vi "Scripting_SaveVi.vi"(7 "ForceResaving(False)":bool, 8 "error in (no error)":errorcluster, 10 "NewPath":path, 11 "VIRefToSaveIn":refnum<vi>) -> (0 "error out":errorcluster, 3 "VIRefToSaveOut":refnum<vi>)   [LabVIEW 2020]
uses:
  SubVIs/GOOP_ProductType.ctl
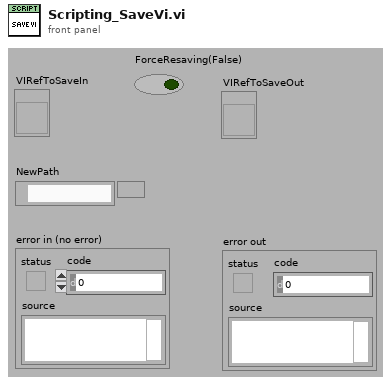
[diagram p1: front panel]
types:
  T1 = typedef "GOOP_ProductType.ctl" = enum16{"InvalidType", "Community Edition", "Professional Edition", "UML Community Edition", "UML Architect Edition"}
  T2 = enum32{"invalid lock state", "Not Locked", "Locked (No Password)", "Password-protected"}
  T3 = enum32{"invalid VI type", "Standard VI", "Control VI", "Global VI", "Polymorphic VI", "Configuration VI", "SubSystem", "Facade VI", "Method VI", "Statechart Diagram VI"}
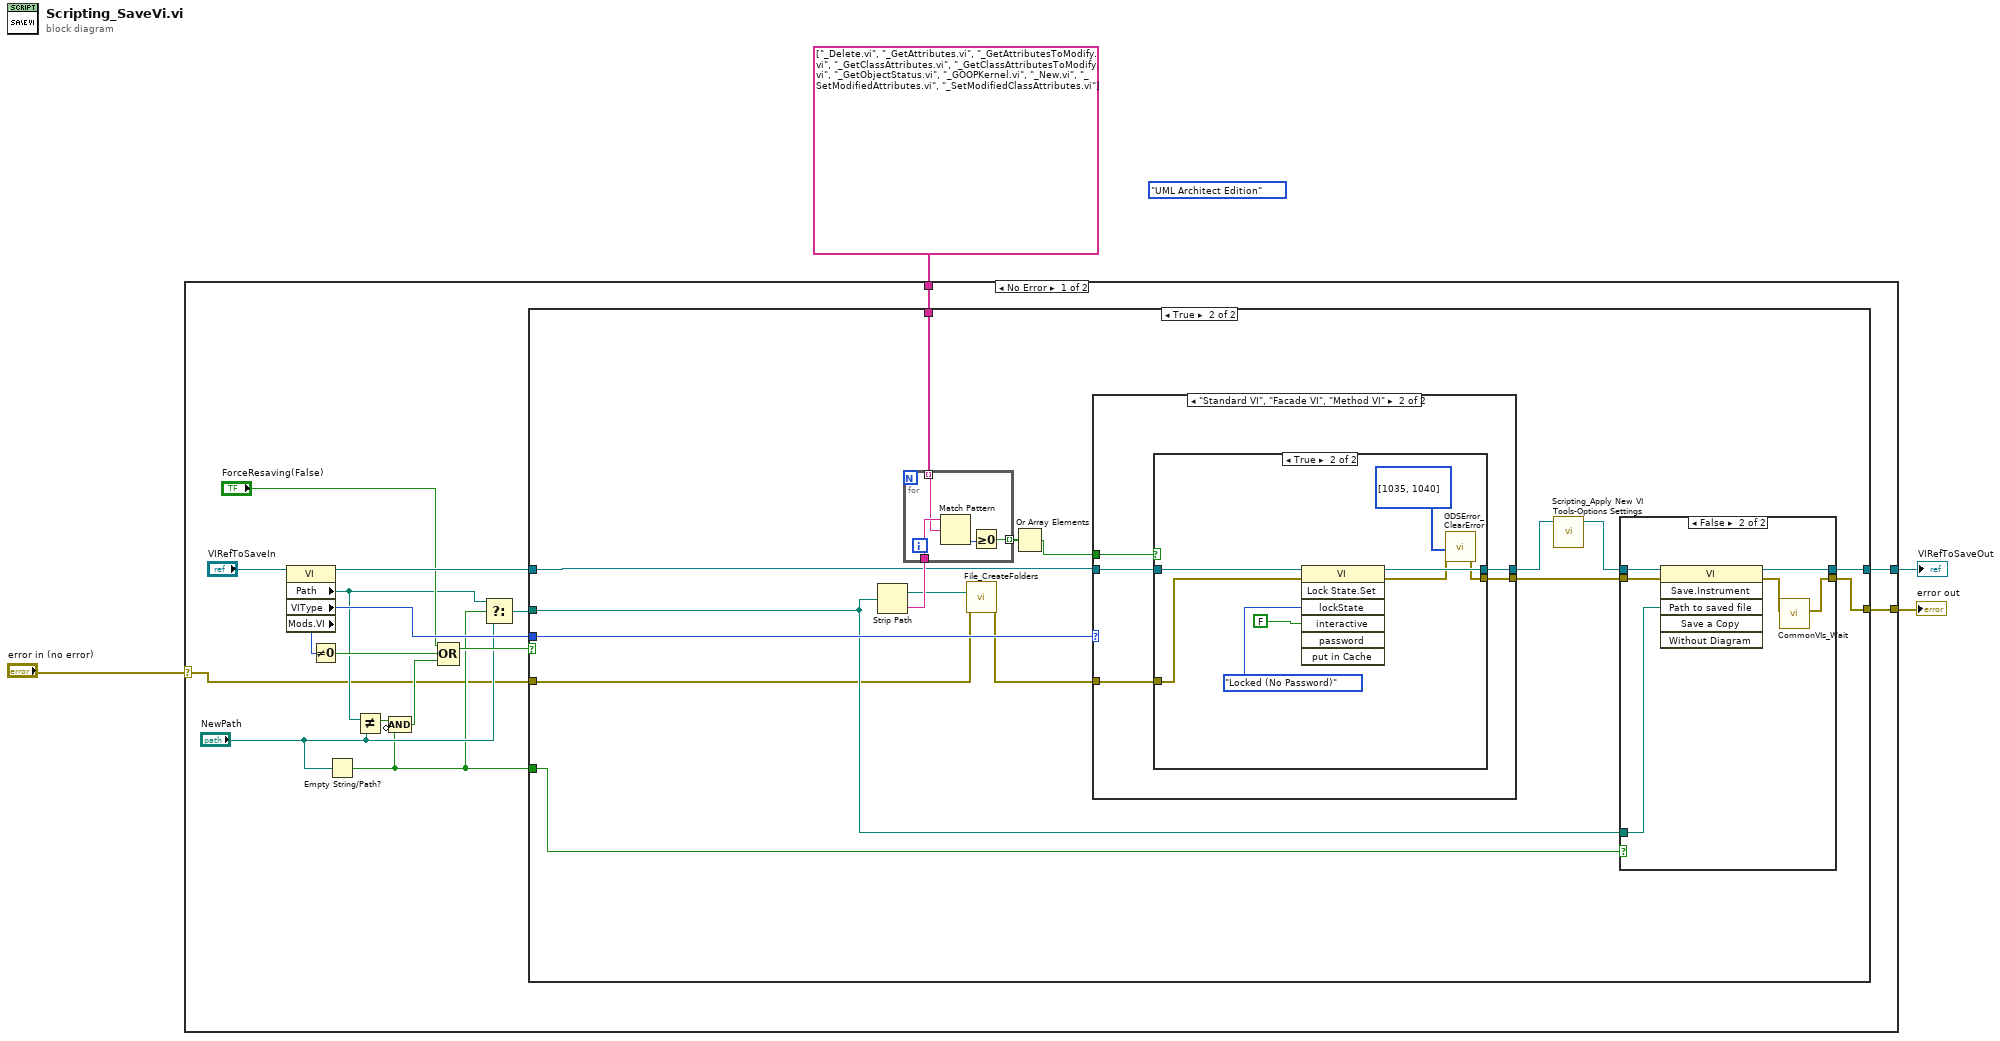
[diagram p0: block diagram]
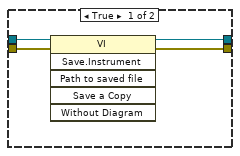
[diagram p3: hidden frame]
diagram:
  (unwired) GOOP_ProductType."UML Architect Edition" ("ProductType")
  n1 = case shown="No Error" "error in (no error)" {
    selector: "error in (no error)" -> [w6 w71]
    tunnel: [w21 w71] -> w4
    tunnel: [w20 _] -> w3
    tunnel: string[] ["_Delete.vi", "_GetAttributes.vi", "_GetAttributesToModify.vi", "_GetClassAttributes.vi", "_GetClassAttributesToModify.vi", "_GetObjectStatus.vi", "_GOOPKernel.vi", "_New.vi", "_SetModifiedAttributes.vi", "_SetModifiedClassAttributes.vi"] ("Array") -> [w5 _]
    frame No Error {
      n2 = property class="VI"(reference="VIRefToSaveIn") -> (reference out=w18:refnum<vi>, "Path"=w10:path, "VIType"=w17:T3, "Mods.VI"=w16:u64)  [unwired: 1 in, 1 out]
      n3 = Not Equal To 0?(x=w16) -> (x != 0?=w15:bool)
      n4 = Empty String/Path?(string/path="NewPath") -> (empty?=w7:bool)
      n5 = Not Equal?(x=w10, y="NewPath") -> (x != y?=w11:bool)
      n6 = Compound Arithmetic op=AND(w11, invert w7) -> (w12:bool)
      n7 = Compound Arithmetic op=OR("ForceResaving(False)", w15, w12) -> (w13:bool)
      n8 = Select(t=w10, s=w7, f="NewPath") -> (s? t:f=w9:path)
      n9 = case shown="True" w13 {
        tunnel: [w22 w39] -> w21
        tunnel: [w23 w38] -> w20
        tunnel: w6 -> [w22 w27]
        tunnel: w18 -> [w23 w30]
        tunnel: w17 -> [_ w36]
        tunnel: w9 -> [_ w33]
        tunnel: w7 -> [_ w35]
        tunnel: w5 -> [_ w34]
        frame False {
        }
        frame True {
          n10 = Strip Path(path=w33) -> (stripped path=w28:path, name=w32:string)
          n11 = for {
            tunnel: w34 -> [w42] mode=indexing
            tunnel: w32 -> [w43]
            tunnel: [w40] -> w31 mode=indexing
            n12 = Match Pattern(string=w43, regular expression=w42) -> (offset past match=w41:i32)  [unwired: 1 in, 3 out]
            n13 = Greater Or Equal To 0?(x=w41) -> (x >= 0?=w40:bool)
          }
          n14 = call "File_CreateFolders.vi"("Path"=w28, "error in (no error)"=w27) -> ("error out"=w26:errorcluster)  [unwired: 15 in, 2 out]
          n15 = Or Array Elements(Boolean array=w31) -> (logical OR=w29:bool)
          n16 = case shown="\"Standard VI\", \"Facade VI\", \"Method VI\"" w36 {
            tunnel: w26 -> [w54 w60]
            tunnel: [w55 w59] -> w25
            tunnel: [w54 w58] -> w37
            tunnel: w30 -> [w55 w57]
            tunnel: w29 -> [_ w56]
            frame Default {
            }
            frame "Standard VI", "Facade VI", "Method VI" {
              n17 = case shown="True" w56 {
                tunnel: w60 -> [w62 w70]
                tunnel: [w61 w69] -> w59
                tunnel: [w62 w66] -> w58
                tunnel: w57 -> [w61 w65]
                frame False {
                }
                frame True {
                  n18 = invoke class="VI" method="Lock State.Set"(reference=w65, error in=w70, "lockState"=T2."Locked (No Password)" ("Lock State"), "interactive"=FALSE ("Interactive")) -> (reference out=w69:refnum<vi>, error out=w67:errorcluster)  [unwired: 3 in, 5 out]
                  n19 = call "GDSError_ClearError.vi"("codes"=i32[] [1035, 1040], "error in (no error)"=w67) -> ("error out"=w66:errorcluster)  [unwired: 16 in, 1 out]
                }
              }
            }
          }
          n20 = call "Scripting_Apply New VI Tools-Options Settings.vi"("VI Refnum"=w25) -> ("dup VI Refnum"=w24:refnum<vi>)  [unwired: 9 in, 1 out]
          n21 = case shown="False" w35 {
            tunnel: [w47 w48] -> w39
            tunnel: [w46 w53] -> w38
            tunnel: w24 -> [w45 w52]
            tunnel: w37 -> [w44 w51]
            tunnel: w33 -> [_ w50]
            frame True {
              n22 = invoke class="VI" method="Save.Instrument"(reference=w45, error in=w44) -> (reference out=w46:refnum<vi>, error out=w47:errorcluster)  [unwired: 4 in, 4 out]
            }
            frame False {
              n23 = invoke class="VI" method="Save.Instrument"(reference=w52, error in=w51, "Path to saved file"=w50) -> (reference out=w53:refnum<vi>, error out=w49:errorcluster)  [unwired: 3 in, 4 out]
              n24 = call "CommonVIs_Wait.vi"("error in"=w49) -> ("error out"=w48:errorcluster)  [unwired: 9 in]
            }
          }
        }
      }
    }
    frame Error {
    }
  }
  "error out" <- w4
  "VIRefToSaveOut" <- w3
